vi "ElectrodeWFM.vi"(5 "Sampling Length":dbl[unit], 7 "Sampling Freq":dbl[unit], 8 "error in (no error)":errorcluster, 9 "Pulse Width Ratio":sgl, 10 "Pulse Amplitude":dbl, 11 "Pulse Freq":dbl[unit]) -> (0 "error out":errorcluster, 1 "Signal Array":dbl[](array[numeric]), 2 "dt [s]":dbl=0.001 format="%0.2p")   [LabVIEW 2012, in "StimulCtrls.lvlib"]
uses:
  StimulCtrls.lvlib
  <vilib>/Analysis/NI_AALBase.lvlib
panel:
  out "Entire Plot":waveform(dbl)(graph)
  out "Electrode Plots":waveform(dbl)[](graph)
  # "Single Pulse"
  # "Entire Signal"
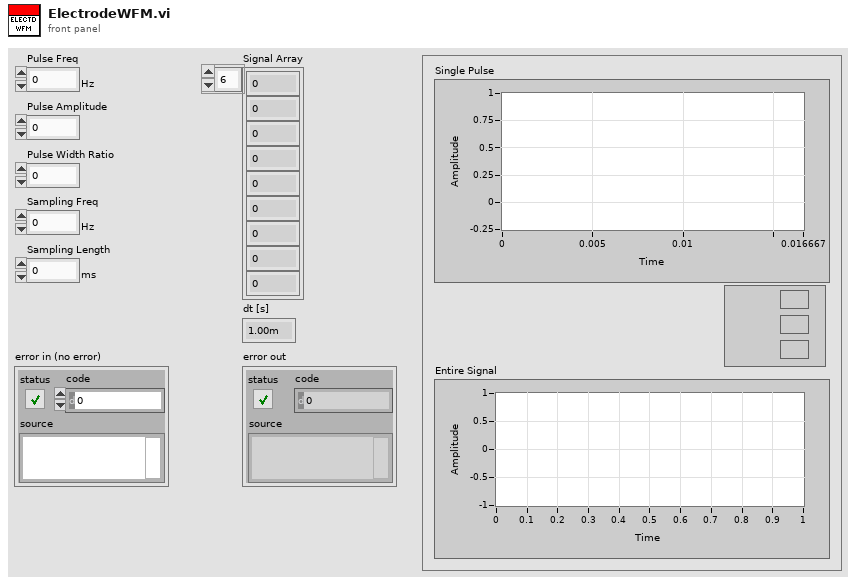
[diagram p1: front panel]
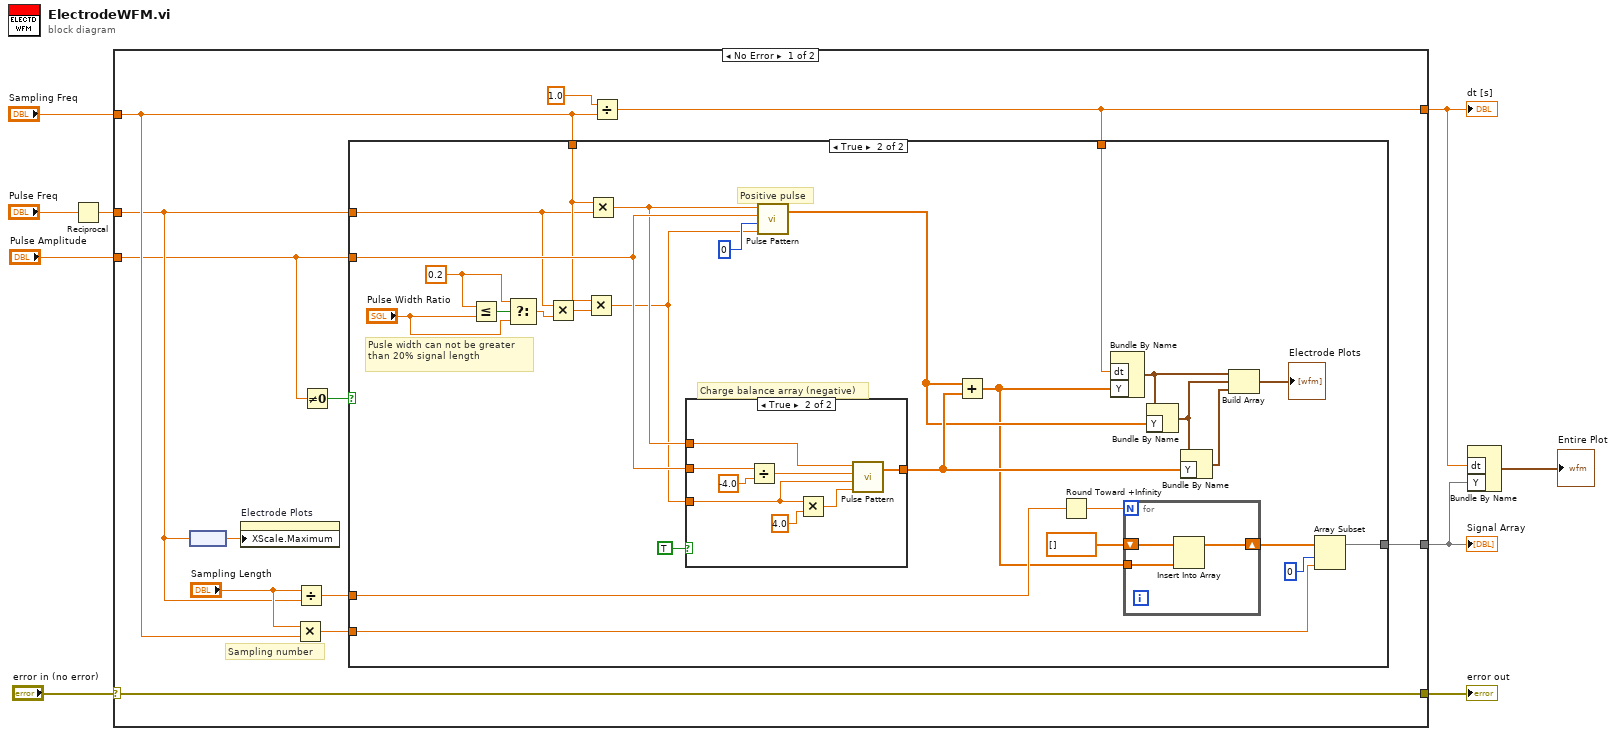
[diagram p0: block diagram]
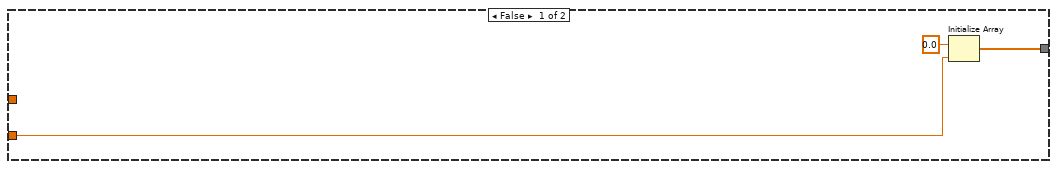
[diagram p2: hidden frame]
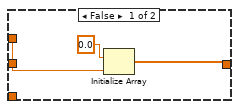
[diagram p3: hidden frame]
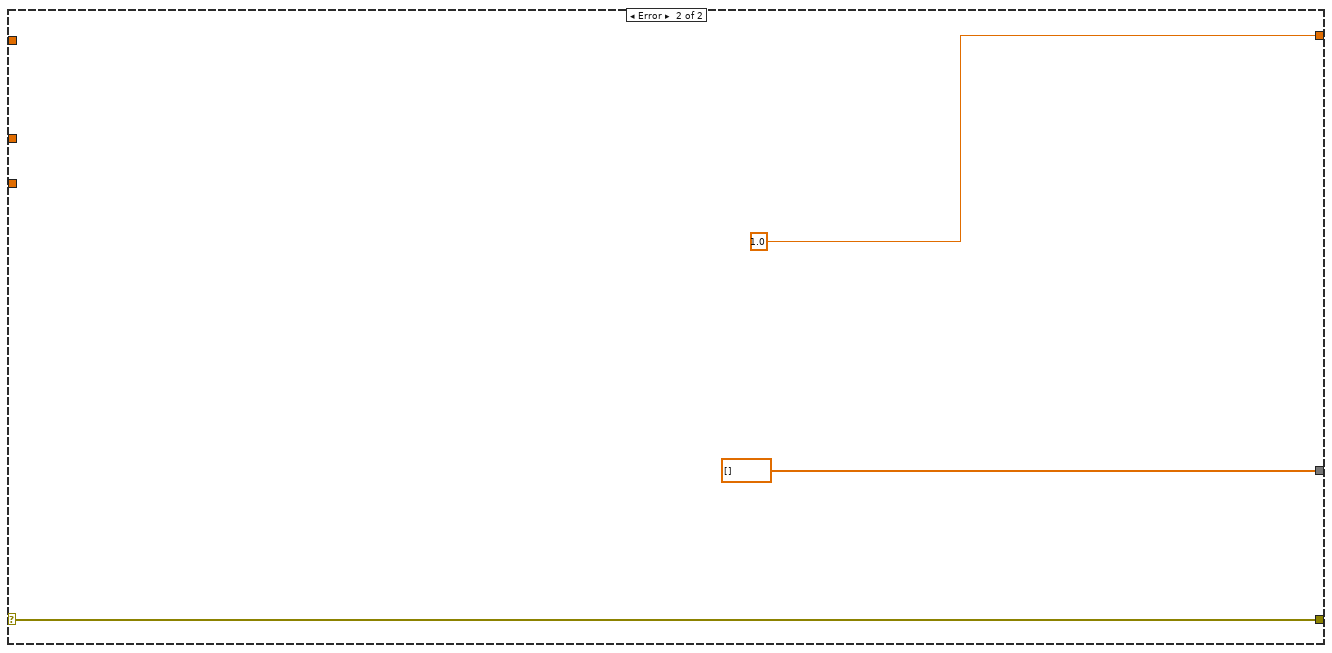
[diagram p4: hidden frame]
diagram:
  n1 = Reciprocal(x="Pulse Freq") -> (1/x=w1:dbl[unit])
  n2 = case shown="No Error" "error in (no error)" {
    selector: "error in (no error)" -> [w21 w68]
    tunnel: [w21 w68] -> w8
    tunnel: [w17 dbl[] [] ("signal")] -> w4
    tunnel: [w20 1.0] -> w3
    tunnel: "Pulse Amplitude" -> [w10 _]
    tunnel: "Sampling Freq" -> [w15 _]
    tunnel: w1 -> [w12 _]
    frame No Error {
      # "Sampling number"
      n3 = node(w12) -> (w13:dbl)
      n4 = property on="Electrode Plots" class="WFGraph (strict)"("XScale.Maximum"=w13) -> ()  [unwired: 2 in, 2 out]
      n5 = Multiply(x="Sampling Length", y=w15) -> (x*y=w14:dbl)
      n6 = Divide(x="Sampling Length", y=w12) -> (x/y=w18:dbl)
      n7 = Not Equal To 0?(x=w10) -> (x != 0?=w11:bool)
      n8 = Divide(x=dbl[unit] 1.0, y=w15) -> (x/y=w20:dbl)
      n9 = case shown="True" w11 {
        tunnel: w10 -> [_ w45]
        tunnel: w20 -> [_ w44]
        tunnel: w18 -> [_ w38]
        tunnel: [w24 w34] -> w17
        tunnel: w15 -> [_ w32]
        tunnel: w14 -> [w23 w31]
        tunnel: w12 -> [_ w25]
        frame False {
          n10 = Initialize Array(0.0 ("element"), w23) -> (w24:dbl[])
        }
        frame True {
          w28 = 0.2
          # "Pusle width can not be greater than 20% signal length"
          # "Charge balance array (negative)"
          # "Positive pulse"
          n11 = Less Or Equal?(x=w28, y="Pulse Width Ratio") -> (x <= y?=w27:bool)
          n12 = Select(t=w28, s=w27, f="Pulse Width Ratio") -> (s? t:f=w29:dbl)
          n13 = Multiply(x=w25, y=w29) -> (x*y=w26:dbl[unit])
          n14 = Multiply(x=w32, y=w26) -> (x*y=w40:dbl)
          n15 = Multiply(x=w32, y=w25) -> (x*y=w43:dbl)
          n16 = case shown="True" TRUE {
            tunnel: w43 -> [w55 w65]
            tunnel: w45 -> [_ w64]
            tunnel: [w56 w61] -> w47
            tunnel: w40 -> [_ w58]
            frame False {
              n17 = Initialize Array(0.0 ("element"), w55) -> (w56:dbl[])
            }
            frame True {
              n18 = Divide(x=w64, y=-4.0) -> (x/y=w63:dbl)
              n19 = Multiply(x=w58, y=4.0) -> (x*y=w59:dbl)
              n20 = call <vilib>:"Pulse Pattern.vi"("width"=w59, "delay"=w58, "amplitude"=w63, "samples"=w65) -> ("Pulse Pattern"=w61:dbl[])  [unwired: 1 out]
            }
          }
          n21 = call <vilib>:"Pulse Pattern.vi"("width"=w40, "delay"=0 ("phase in"), "amplitude"=w45, "samples"=w43) -> ("Pulse Pattern"=w46:dbl[])  [unwired: 1 out]
          n22 = Add(x=w46, y=w47) -> (x+y=w36:dbl[])
          n23 = Round Toward +Infinity(x=w38) -> (ceil(x): smallest int >= x=w37:dbl)
          n24 = Bundle By Name("dt"=w44, "Y"=w36) -> (w50:waveform(dbl))  [unwired: 1 in]
          n25 = for {
            N: w37 -> [_]
            shift-right: [w52] -> w39
            shift-left: dbl[] [] -> [w54]
            tunnel: w36 -> [w53]
            n26 = Insert Into Array(array=w54, new element=w53) -> (w52:dbl[])  [unwired: 1 in]
          }
          n27 = Bundle By Name(cluster=w50, "Y"=w46) -> (w49:waveform(dbl))
          n28 = Bundle By Name(cluster=w49, "Y"=w47) -> (w48:waveform(dbl))
          n29 = Build Array(w50, w49, w48) -> (→"Electrode Plots":waveform(dbl)[])
          n30 = Array Subset(array=w39, index=0, length=w31) -> (w34:dbl[])
        }
      }
    }
    frame Error {
    }
  }
  "error out" <- w8
  "Signal Array" <- w4
  "dt [s]" <- w3
  n31 = Bundle By Name("dt"=w3, "Y"=w4) -> (→"Entire Plot":waveform(dbl))  [unwired: 1 in]
